vi "PH_IEEE1394Camera.set Visibility of Cam Attribute Value Set Knobs.vi"(0 "VI in":refnum<vi>, 2 "Index of selected Attribute":u32, 5 "error in (no error)":errorcluster) -> (14 "VI out":refnum<vi>, 19 "error out":errorcluster)   [LabVIEW 2014, in "PH_IEEE1394Camera.lvlib"]
uses:
  PH_IEEE1394Camera.lvlib
  PH_Basics/PH_Common/PH_Common.lvlib
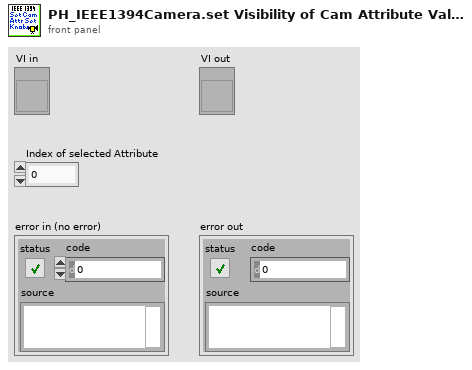
[diagram p1: front panel]
types:
  T1 = typedef "PH_IEEE1394Camera.lvlib/PH_IEEE1394Camera.i attribute.ctl" = cluster{"Gui Refs":cluster{"Brightness":refnum<vi>, "Shutter":refnum<vi>, "Gain":refnum<vi>, "Center of Gravity":refnum<vi>, "Supported Video Modes":refnum<vi>, "Trigger Polarity":refnum<vi>, "Trigger Mode":refnum<vi>, "Trigger Timeout":refnum<vi>, "Bit Depth":refnum<vi>, "Video Mode":refnum<vi>, "Top":refnum<vi>, "Bottom":refnum<vi>, "Left":refnum<vi>, "Right":refnum<vi>, "Set ROI to Maximum":refnum<vi>, "Camera Details":refnum<vi>, "Current Cam Attributes":refnum<vi>, "Attribute to set":refnum<vi>, "Num Value":refnum<vi>, "String Value":refnum<vi>, "Bool Value":refnum<vi>, "Set Cam Attribute":refnum<vi>}, "Cam":cluster{"IMAQ1394 Session":T2, "Camera Details":T3}, "Current Attributes":T4[], "Supported Video Modes ":cluster{"Video Mode":u32, "Video Mode Name":string}[], "Wanted Attributes":cluster{"Name":string, "Num Value":dbl, "String Value":string, "Boolean Value":bool}[], "Cam Attributes":T6}
  T2 = typedef "IMAQdx.ctl" = refnum<k21>
  T3 = typedef "PH_IEEE1394Camera.lvlib/PH_IEEE1394Camera.Cam Details.ctl" = cluster{"Model":string, "Serial Number":dbl, "Cam name (Machinery)":string, "Bus Type":string}
  T4 = typedef "PH_IEEE1394Camera.lvlib/PH_IEEE1394Camera.Cam Attribute.ctl" = cluster{"Information":cluster{"Type":T5, "Readable":bool, "Writable":bool, "Name":string}, "Num Value":dbl, "String Value":string, "Maximum":dbl, "Minimum":dbl, "Units":string, "Description":string, "EnumStrings[]":string[], "EnumValues[]":u32[], "Boolean Value":bool}
  T5 = typedef "NI_Vision_Acquisition_Software.lvlib/IMAQdx Attribute Type.ctl" = enum32{"U32", "I64", "DBL", "String", "Enum", "Bool", "Command"}
  T6 = typedef "PH_IEEE1394Camera.lvlib/PH_IEEE1394Camera.Relevant Cam Attributes.ctl" = cluster{"Video Mode":cluster{"Name":string, "Index":i32}, "Brightness":cluster{"Name":string, "Index":i32}, "Gain":cluster{"Name":string, "Index":i32}, "Shutter":cluster{"Name":string, "Index":i32}, "Trigger Pol":cluster{"Name":string, "Index":i32}, "Trigger Mode":cluster{"Name":string, "Index":i32}, "Timeout":cluster{"Name":string, "Index":i32}, "Bit Depth":cluster{"Name":string, "Index":i32}, "Pixel Bits":cluster{"Name":string, "Index":i32}, "Pixel Bytes":cluster{"Name":string, "Index":i32}, "Left":cluster{"Name":string, "Index":i32}, "Right":cluster{"Name":string, "Index":i32}, "Top":cluster{"Name":string, "Index":i32}, "Bottom":cluster{"Name":string, "Index":i32}}
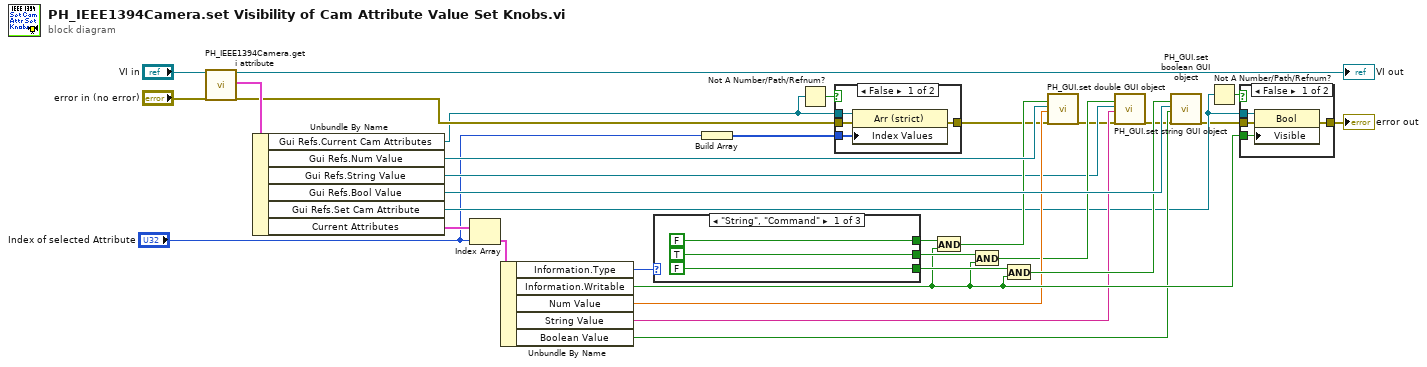
[diagram p0: block diagram]
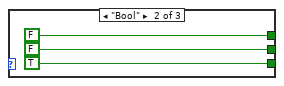
[diagram p4: hidden frame]
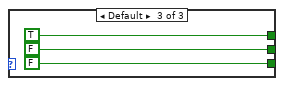
[diagram p5: hidden frame]
diagram:
  n1 = call "PH_IEEE1394Camera.get i attribute.vi"("i ref in"="VI in", "error in (no error)"="error in (no error)") -> ("i ref out"=→"VI out":refnum<vi>, "i attribute"=w26:T1, "error out"=w6:errorcluster)  [unwired: 15 in]
  n2 = Unbundle By Name(w26) -> ("Gui Refs.Current Cam Attributes"=w2:refnum<vi>, "Gui Refs.Num Value"=w16:refnum<vi>, "Gui Refs.String Value"=w11:refnum<vi>, "Gui Refs.Bool Value"=w19:refnum<vi>, "Gui Refs.Set Cam Attribute"=w10:refnum<vi>, "Current Attributes"=w27:T4[])
  n3 = Index Array(array=w27, index="Index of selected Attribute") -> (element=w28:T4)
  n4 = Unbundle By Name(w28) -> ("Information.Type"=w29:T5, "Information.Writable"=w21:bool, "Num Value"=w15:dbl, "String Value"=w12:string, "Boolean Value"=w17:bool)
  n5 = case shown="\"String\", \"Command\"" w29 {
    tunnel: [FALSE FALSE TRUE] -> w30
    tunnel: [TRUE FALSE FALSE] -> w31
    tunnel: [FALSE TRUE FALSE] -> w32
    frame "String", "Command" {
    }
    frame "Bool" {
    }
    frame Default {
    }
  }
  n6 = Build Array("Index of selected Attribute") -> (w1:u32[])
  n7 = Not A Number/Path/Refnum?(number/path/refnum=w2) -> (NaN/Path/Refnum?=w4:bool)
  n8 = case shown="False" w4 {
    tunnel: w6 -> [w45 w46]
    tunnel: [w44 w46] -> w5
    tunnel: w2 -> [w43 _]
    tunnel: w1 -> [w42 _]
    frame False {
      n9 = property on="Property Node" class="Arr (strict)"(reference=w43, error in=w45, "Index Values"=w42) -> (error out=w44:errorcluster)  [unwired: 1 out]
    }
    frame True {
    }
  }
  n10 = And(x=w30, y=w21) -> (x .and. y?=w14:bool)
  n11 = And(x=w31, y=w21) -> (x .and. y?=w13:bool)
  n12 = And(x=w32, y=w21) -> (x .and. y?=w18:bool)
  n13 = call "PH_GUI.set double GUI object.vi"("visible (true)"=w14, "GUI object Ref"=w16, "value"=w15, "error in (no error)"=w5) -> ("error out"=w9:errorcluster)  [unwired: 15 in]
  n14 = call "PH_GUI.set string GUI object.vi"("Visible (True)"=w13, "GUI object Ref"=w11, "Text"=w12, "error in"=w9) -> ("error out"=w8:errorcluster)  [unwired: 15 in]
  n15 = call "PH_GUI.set boolean GUI object.vi"("Visible (true)"=w18, "Boolean Knob GUI Ref"=w19, "Value"=w17, "error in (no error)"=w8) -> ("error out"=w7:errorcluster)  [unwired: 15 in]
  n16 = Not A Number/Path/Refnum?(number/path/refnum=w10) -> (NaN/Path/Refnum?=w22:bool)
  n17 = case shown="False" w22 {
    tunnel: w21 -> [w50 _]
    tunnel: w7 -> [w49 w51]
    tunnel: [w48 w51] -> w20
    tunnel: w10 -> [w47 _]
    frame False {
      n18 = property on="Property Node" class="Bool"(reference=w47, error in=w49, "Visible"=w50) -> (error out=w48:errorcluster)  [unwired: 1 out]
    }
    frame True {
    }
  }
  "error out" <- w20
